vi "unwarp phase.vi"(9 "zero!":bool, 11 "phase in (0..4096)":dbl[](array[numeric])=[0.0, 0.0, 0.0]) -> (3 "unwrapped phase out (rad)":dbl[](array[numeric]))   [LabVIEW 2018]
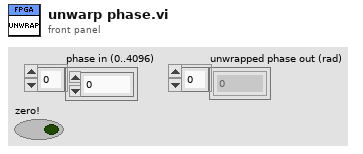
[diagram p1: front panel]
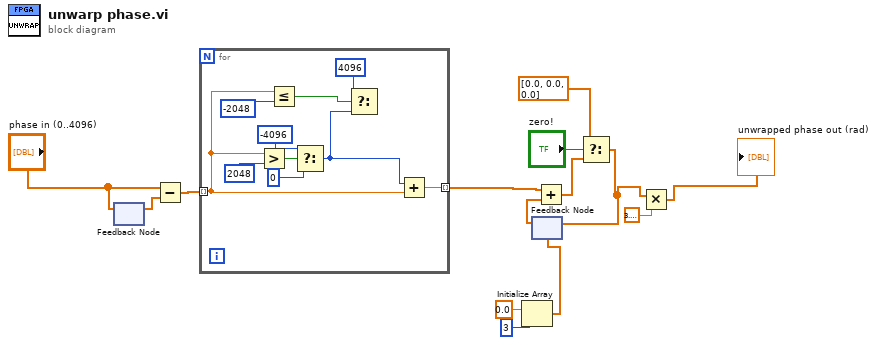
[diagram p0: block diagram]
diagram:
  n1 = feedback #1() -> (w11:dbl[])  [unwired: 1 in]
  n2 = feedback-in #1("phase in (0..4096)") -> ()
  n3 = Subtract(x="phase in (0..4096)", y=w11) -> (x-y=w14:dbl[])
  n4 = for {
    tunnel: w14 -> [w17] mode=indexing
    tunnel: [w15] -> w10 mode=indexing
    n5 = Greater?(x=w17, y=2048) -> (0:w23:bool)
    n6 = Less Or Equal?(x=w17, y=-2048) -> (x <= y?=w20:bool)
    n7 = Select(t=-4096, s=w23, f=0) -> (s? t:f=w16:i32)
    n8 = Select(t=4096, s=w20, f=w16) -> ()  [unwired: 1 out]
    n9 = Add(x=w16, y=w17) -> (x+y=w15:dbl)
  }
  n10 = Initialize Array(0.0 ("element"), 3 ("dimension size")) -> (w1:dbl[])
  n11 = feedback #2(w1) -> (w12:dbl[])
  n12 = Add(x=w10, y=w12) -> (x+y=w6:dbl[])
  n13 = Select(t=dbl[] [0.0, 0.0, 0.0], s="zero!", f=w6) -> (s? t:f=w5:dbl[])
  n14 = feedback-in #2(w5) -> ()
  n15 = Multiply(x=w5, y=3.141592653589793) -> (x*y=→"unwrapped phase out (rad)":dbl[])
